vi "Main.vi"() -> ()   [LabVIEW 2014]
doc: "The myRIO Project template acquires acceleration data from the onboard accelerometer and displays the changes of acceleration values in a waveform chart."
uses:
  C:/Program Files (x86)/National Instruments/LabVIEW 2014/examples/robotics/Vision/Color Tracking/HueSlider.ctl
  <vilib>/myRIO/Instrument Drivers/Onboard IO/AI/typedefs/AI Reference.ctl
  <vilib>/myRIO/Common/Instrument Driver Framework/Utilities/typedefs/myRIO Generic Hardware Reference.ctl
  <vilib>/myRIO/Common/Instrument Driver Framework/Utilities/typedefs/Hardware Version Enum.ctl
  <vilib>/myRIO/Common/Instrument Driver Framework/Utilities/typedefs/myRIO v1.0 Reference.ctl
  <vilib>/myRIO/Common/Instrument Driver Framework/Utilities/typedefs/Generic FPGA Reference.ctl
  <vilib>/myRIO/Common/Instrument Driver Framework/myRIO v1.0/AI/typedefs/AI Channels List.ctl
  <vilib>/myRIO/Common/Instrument Driver Framework/myRIO v1.0/AI/typedefs/AI Channels Enum.ctl
  <vilib>/myRIO/Common/Instrument Driver Framework/Utilities/typedefs/Analog Scaling Constants List.ctl
  <vilib>/myRIO/Common/Instrument Driver Framework/Utilities/typedefs/Analog Scaling Constants.ctl
  <vilib>/userdefined/High Color/nirio_resource_hc.ctl
  <vilib>/myRIO/Instrument Drivers/Onboard IO/PWM/typedefs/PWM Reference.ctl
  <vilib>/myRIO/Common/Instrument Driver Framework/myRIO v1.0/PWM/typedefs/PWM Channels Enum.ctl
  <vilib>/myRIO/Instrument Drivers/Onboard IO/PWM/typedefs/PWM Configuration.ctl
  <vilib>/myRIO/Instrument Drivers/Onboard IO/DIO/typedefs/DIO Reference.ctl
  <vilib>/myRIO/Common/Instrument Driver Framework/myRIO v1.0/DIO/typedefs/DIO Channels List.ctl
  <vilib>/myRIO/Common/Instrument Driver Framework/myRIO v1.0/DIO/typedefs/DIO Channels Enum.ctl
  <vilib>/myRIO/Common/Instrument Driver Framework/myRIO v1.0/Encoder/typedefs/Encoder Signal Mode.ctl
  <vilib>/myRIO/Instrument Drivers/Onboard IO/Encoder/typedefs/Encoder Reference.ctl
  <vilib>/myRIO/Common/Instrument Driver Framework/myRIO v1.0/Encoder/typedefs/Encoder Channels Enum.ctl
  <vilib>/myRIO/Common/Instrument Driver Framework/myRIO v1.0/Encoder/typedefs/Encoder Configuration v1.0.ctl
  <vilib>/myRIO/Common/Instrument Driver Framework/Utilities/vis/Is FPGA Ref Available.vi
  <vilib>/myRIO/Common/Instrument Driver Framework/myRIO v1.0/AI/vis/myRIO v1.1 Open AI.vi
  <vilib>/myRIO/Instrument Drivers/Onboard IO/AI/vis/Read.vi
  <vilib>/myRIO/Common/Instrument Driver Framework/myRIO v1.0/PWM/vis/myRIO v1.1 Open PWM.vi
  <vilib>/myRIO/Instrument Drivers/Onboard IO/PWM/vis/Set Duty Cycle and Frequency.vi
  <vilib>/myRIO/Common/Instrument Driver Framework/myRIO v1.0/Encoder/vis/myRIO v1.1 Open Encoder.vi
  <vilib>/myRIO/Instrument Drivers/Onboard IO/Encoder/vis/Read.vi
  <vilib>/myRIO/Common/Instrument Driver Framework/myRIO v1.0/DIO/vis/myRIO v1.1 Open DIO.vi
  <vilib>/myRIO/Instrument Drivers/Onboard IO/DIO/vis/Write.vi
  <vilib>/myRIO/Common/Instrument Driver Framework/Utilities/vis/Validate Channels.vi
  <vilib>/myRIO/Common/Instrument Driver Framework/myRIO v1.0/AI/vis/myRIO v1.0 Reserve AI.vi
  <vilib>/myRIO/Common/Instrument Driver Framework/myRIO v1.0/PWM/vis/myRIO v1.0 Reserve PWM.vi
  <vilib>/myRIO/Common/Instrument Driver Framework/myRIO v1.0/Encoder/vis/myRIO v1.0 Reserve Encoder.vi
  <vilib>/myRIO/Common/Instrument Driver Framework/myRIO v1.0/DIO/vis/myRIO v1.0 Reserve DIO.vi
  <vilib>/myRIO/Common/Instrument Driver Framework/myRIO v1.0/UART/vis/myRIO v1.0 Close UART.vi
  <vilib>/myRIO/Common/Instrument Driver Framework/myRIO v1.0/AI/vis/myRIO v1.0 Build MUX Configuration AI.vi
  <vilib>/myRIO/Common/Instrument Driver Framework/myRIO v1.0/Resource Manager/vis/myRIO v1.0 Reserve Channel List.vi
  <vilib>/myRIO/Common/Instrument Driver Framework/myRIO v1.0/PWM/vis/myRIO v1.0 Build MUX Configuration PWM.vi
  <vilib>/myRIO/Common/Instrument Driver Framework/myRIO v1.0/Encoder/vis/myRIO v1.0 Build MUX Configuration Encoder.vi
  <vilib>/myRIO/Common/Instrument Driver Framework/myRIO v1.0/DIO/vis/myRIO v1.0 Build MUX Configuration DIO.vi
  <vilib>/myRIO/Common/Instrument Driver Framework/myRIO v1.0/Resource Manager/vis/myRIO v1.0 Reserve Channel.vi
  <vilib>/myRIO/Common/Instrument Driver Framework/myRIO v1.0/Resource Manager/vis/myRIO v1.0 Unreserve Channel.vi
  <vilib>/myRIO/Common/Instrument Driver Framework/myRIO v1.0/Resource Manager/vis/myRIO v1.0 Create Configuration List.vi
  <vilib>/myRIO/Common/Instrument Driver Framework/myRIO v1.0/Resource Manager/vis/myRIO v1.0 Build Mutex Name.vi
  <vilib>/Utility/VariantDataType/GetNumericInfo.vi
  <vilib>/Utility/error.llb/Error Cluster From Error Code.vi
  <vilib>/myRIO/Common/Instrument Driver Framework/myRIO v1.0/myRIO v1.1 Open.vi
  <vilib>/myRIO/Common/Instrument Driver Framework/myRIO v1.0/AI/vis/myRIO v1.0 Get Scaling Constants AI.vi
  <vilib>/myRIO/Common/Instrument Driver Framework/Utilities/vis/IO Manager.vi
  <vilib>/myRIO/Common/Instrument Driver Framework/Utilities/vis/Configuration Manager.vi
  <vilib>/myRIO/Common/Instrument Driver Framework/myRIO v1.0/myRIO v1.0 Close.vi
  <vilib>/myRIO/Common/Instrument Driver Framework/myRIO v1.0/AI/vis/myRIO v1.0 Read AI.vi
  <vilib>/myRIO/Common/Instrument Driver Framework/myRIO v1.0/Resource Manager/vis/myRIO v1.0 Configure IO.vi
  <vilib>/myRIO/Common/Instrument Driver Framework/myRIO v1.0/PWM/vis/myRIO v1.0 Write PWM.vi
  <vilib>/myRIO/Common/Instrument Driver Framework/myRIO v1.0/DIO/vis/myRIO v1.0 Write DIO.vi
  <vilib>/myRIO/Common/Instrument Driver Framework/myRIO v1.0/Encoder/vis/myRIO v1.0 Configure Encoder.vi
  <vilib>/myRIO/Common/Instrument Driver Framework/myRIO v1.0/Encoder/vis/myRIO v1.0 Read Encoder.vi
  <vilib>/myRIO/Common/Instrument Driver Framework/Utilities/vis/FPGA Ref Manager.vi
  <vilib>/myRIO/Common/Instrument Driver Framework/myRIO v1.0/myRIO v1.0 Reset FPGA.vi
  <vilib>/myRIO/Common/Instrument Driver Framework/myRIO v1.0/IRQ/vis/myRIO v1.0 IRQ Info FGV.vi
  <vilib>/myRIO/Common/Instrument Driver Framework/myRIO v1.0/IRQ/vis/myRIO v1.0 Timer IRQ Info FGV.vi
  <vilib>/myRIO/Common/Instrument Driver Framework/myRIO v1.0/IRQ/vis/myRIO v1.0 ISR Agent.vi
  <vilib>/myRIO/Express VI/Onboard IO/AI/AI Express VI.xnode
  <vilib>/myRIO/Instrument Drivers/Onboard IO/AI/vis/myRIO AI Open.xnode
  <vilib>/myRIO/Express VI/Onboard IO/PWM/PWM Express VI.xnode
  <vilib>/myRIO/Instrument Drivers/Onboard IO/PWM/vis/myRIO PWM Open.xnode
  <vilib>/myRIO/Express VI/Onboard IO/DO/DO Express VI.xnode
  <vilib>/myRIO/Instrument Drivers/Onboard IO/DIO/vis/myRIO DIO Open.xnode
  <vilib>/myRIO/Express VI/Onboard IO/Encoder/Encoder Express VI.xnode
  <vilib>/myRIO/Instrument Drivers/Onboard IO/Encoder/vis/myRIO Encoder Open.xnode
  <vilib>/myRIO/Instrument Drivers/Utilities/Utilities.lvlib
  <vilib>/myRIO/Instrument Drivers/Onboard IO/PWM/PWM.lvlib
  <vilib>/myRIO/Instrument Drivers/Onboard IO/DIO/DIO.lvlib
  <vilib>/myRIO/Instrument Drivers/Onboard IO/Encoder/Encoder.lvlib
  <vilib>/vision/driver/NI_Vision_Acquisition_Software.lvlib
  <vilib>/vision/NI_Vision_Development_Module.lvlib
  <vilib>/myRIO/Instrument Drivers/Onboard IO/AI/AI.lvlib
  <vilib>/Analysis/NI_AALPro.lvlib
  <vilib>/Analysis/NI_AALBase.lvlib
panel:
  out "LCD display":string
  in  "Samples":i32=128
  in  "Amplitude":dbl=5.0 format="%#.6g"
  in  "Width (samples)":i32=32
  in  "Delay (samples)":i32=64
  in  "Filter rank":i32(slide)=7 scale=0.0..30.0
  in  "Gaussian noise sigma":dbl(slide)=0.8 scale=0.0..2.0
  out "Waveform Graph":dbl[][](graph)
  out "Width (est)":dbl format="%#.2g"
  out "Delay (est)":dbl format="%#.2g"
  out "Amplitude (est)":dbl format="%#.2g"
  in  "seed":i32=-1
  out "Gauss 1 fit":cluster{"a":dbl, "m":dbl, "sigma":dbl}
  out "Gauss 2 fit":cluster{"a":dbl, "m":dbl, "sigma":dbl}
  out "Gauss 3 fit":cluster{"a":dbl, "m":dbl, "sigma":dbl}
  out "DC offset fit":dbl
  out "웨이브폼 차트":dbl(graph)
  out "C/AI0 (C/AI0 (AI0))":dbl
  out "Image 2":T1(plugin-control)
  in  "Speed\n(PWM Duty %) 2":dbl(slide)=1.0
  in  "Hue range":T2={"Min"=232, "Max"=21} scale=0.0..255.0
  in  "Stop 2":bool
  out "Image":T1(plugin-control)
  in  "Camera Name":refnum<k21>="cam3" caption="IMAQdx Session"
  in  "Reset Counter":bool
  out "Counter Value":i32
  out "Counter Direction":enum16{"Counting Up", "Counting Down"}(ring)
  in  "Direction":bool
  in  "Speed\n(PWM Duty %)":dbl(slide)=1.0
  out "error out":errorcluster
  in  "Stop":bool
  # "Control Motor"
  # "Read Encoder"
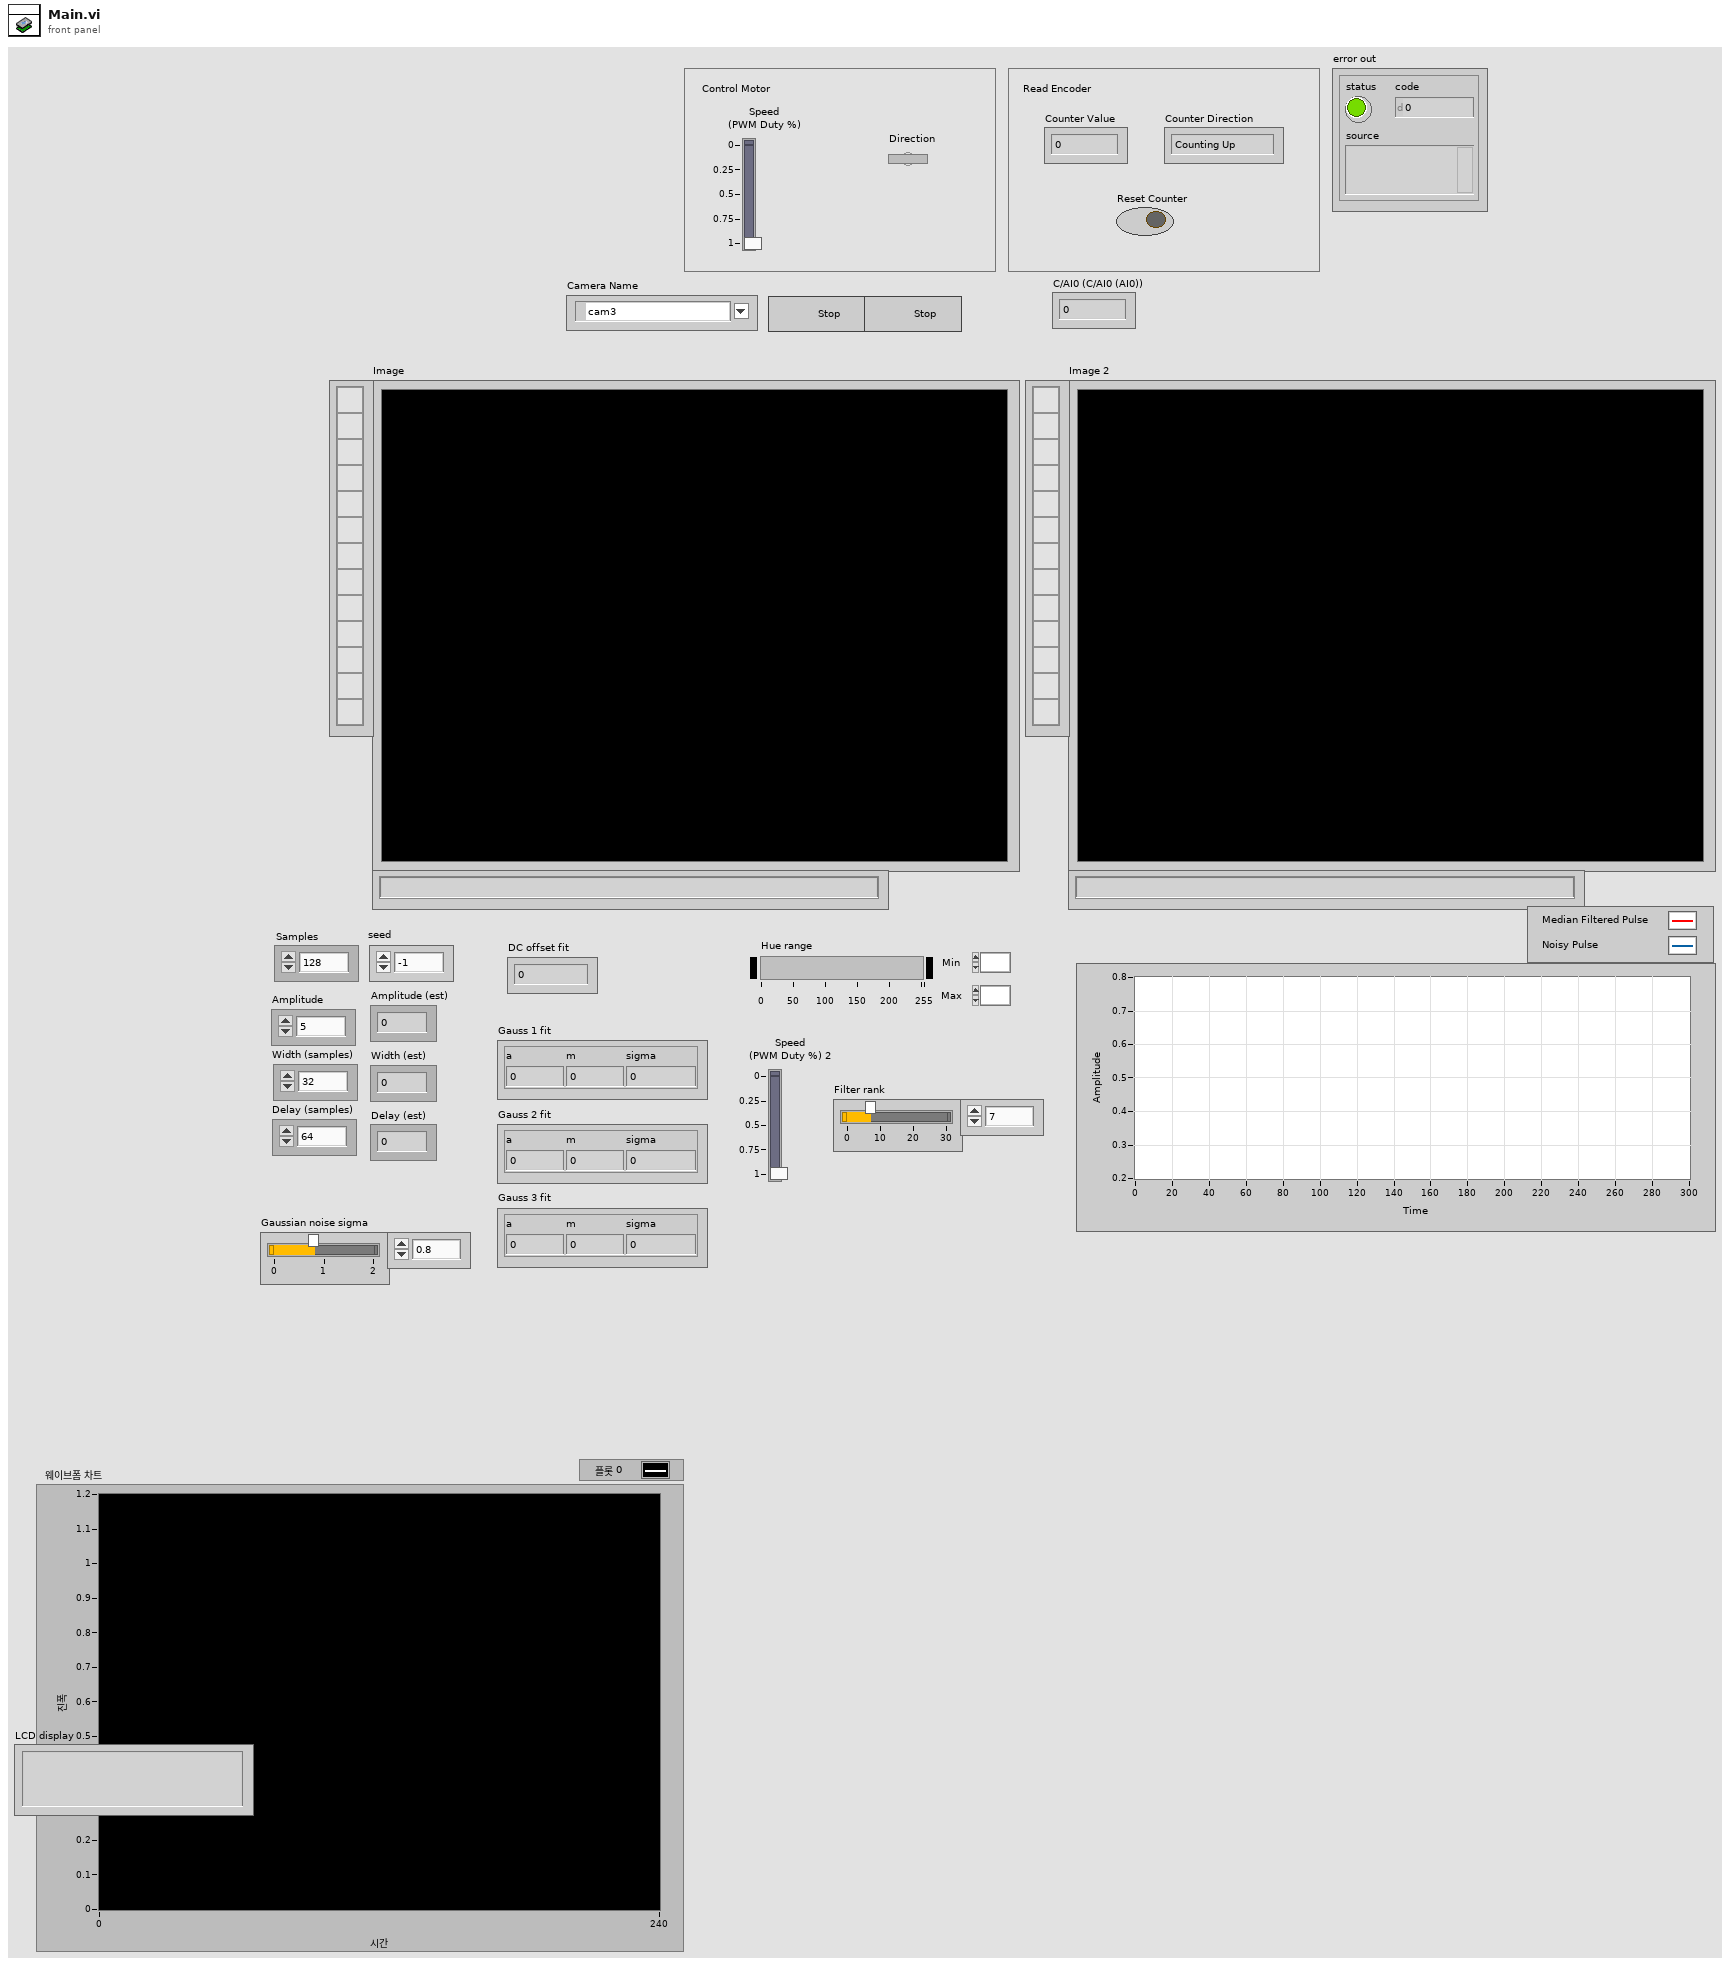
[diagram p1: front panel]
types:
  T1 = typedef "IMAQ Image.ctl" = refnum<image>
  T2 = typedef "HueSlider.ctl" = cluster{"Min":i32, "Max":i32}
  T3 = typedef "IMAQ Circle" = cluster{"Center X":i32, "Center Y":i32, "Inner Radius":i32, "Outer Radius":i32, "Start Angle":dbl, "End Angle":dbl}
  T4 = typedef "AI.lvlib/AI Reference.ctl" = cluster{"myRIO Reference":T5, "AI Channels List":T9, "AI Scaling Constants List":T11}
  T5 = typedef "myRIO Generic Hardware Reference.ctl" = cluster{"myRIO Model":T6, "myRIO Hardware Reference":T7}
  T6 = typedef "Hardware Version Enum.ctl" = enum16{"Unknown", "myRIO-1900", "myRIO-1950"}
  T7 = typedef "myRIO v1.0 Reference.ctl" = cluster{"Generic FPGA Reference":T8, "Allow multiple opens":bool}
  T8 = typedef "Generic FPGA Reference.ctl" = refnum<k20>
  T9 = typedef "AI Channels List.ctl" = T10[]
  T10 = typedef "AI Channels Enum.ctl" = enum16{"Not Connected", "AudioIn/Left", "AudioIn/Right", "C/AI0", "C/AI1", "A/AI0", "A/AI1", "A/AI2", "A/AI3", "B/AI0", "B/AI1", "B/AI2", "B/AI3"}
  T11 = typedef "Analog Scaling Constants List.ctl" = T12[]
  T12 = typedef "Analog Scaling Constants.ctl" = cluster{"LSB Weight (Volts)":dbl, "Offset (Volts)":dbl, "Signed?":bool}
  T13 = typedef "nirio_resource_hc.ctl" = tag
  T14 = typedef "IMAQ Rectangle" = cluster{"Left":i32, "Top":i32, "Right":i32, "Bottom":i32, "Rotation":dbl}
  T15 = typedef "PWM.lvlib/PWM Reference.ctl" = cluster{"myRIO Reference":T5, "PWM Channels Enum":T16, "PWM Configuration":T17}
  T16 = typedef "PWM Channels Enum.ctl" = enum16{"Not Connected", "C/PWM0", "C/PWM1", "A/PWM0", "A/PWM1", "A/PWM2", "B/PWM0", "B/PWM1", "B/PWM2"}
  T17 = typedef "PWM.lvlib/PWM Configuration.ctl" = cluster{"Frequency":dbl, "Duty Cycle":dbl}
  T18 = typedef "Encoder.lvlib/Encoder Reference.ctl" = cluster{"myRIO Reference":T5, "Encoder Channels Enum":T19}
  T19 = typedef "Encoder Channels Enum.ctl" = enum16{"Not Connected", "C/ENC0", "C/ENC1", "A/ENC", "B/ENC"}
  T20 = typedef "Encoder Signal Mode.ctl" = enum16{"Quadrature phase signal", "Step and direction signal"}
  T21 = typedef "DIO.lvlib/DIO Reference.ctl" = cluster{"myRIO Reference":T5, "DIO Channels List":T22}
  T22 = typedef "DIO Channels List.ctl" = T23[]
  T23 = typedef "DIO Channels Enum.ctl" = enum16{"Not Connected", "C/DIO0", "C/DIO1", "C/DIO2", "C/DIO3", "C/DIO4", "C/DIO5", "C/DIO6", "C/DIO7", "A/DIO0", "A/DIO1", "A/DIO2", "A/DIO3", "A/DIO4", "A/DIO5", "A/DIO6", "A/DIO7", "A/DIO8", "A/DIO9", "A/DIO10", "A/DIO11", "A/DIO12", "A/DIO13", "A/DIO14", "A/DIO15", "B/DIO0", "B/DIO1", "B/DIO2", "B/DIO3", "B/DIO4", "B/DIO5", "B/DIO6", "B/DIO7", "B/DIO8", "B/DIO9", "B/DIO10", "B/DIO11", "B/DIO12", "B/DIO13", "B/DIO14", "B/DIO15", "LED0", "LED1", "LED2", "LED3", "Button0"}
  T24 = typedef "IMAQdx.ctl" = refnum<k21>
  T25 = cluster{"Global Rectangle":i32[], "Contours":cluster{"Contour Type":u32, "ROI Type":u32, "Points":i32[]}[]}
  T26 = cluster{"Center":cluster{"X":sgl, "Y":sgl}, "Radius":dbl}
  T27 = typedef "ROI Descriptor" = cluster{"Global Rectangle":i32[], "Contours":cluster{"ID":enum32{"External", "Internal"}, "Type":u32, "Coordinates":i32[]}[]}
  T28 = cluster{"Area":dbl, "Number of Holes":dbl, "Bounding Rect":cluster{"Left":dbl, "Top":dbl, "Right":dbl, "Bottom":dbl}, "Center of Mass":cluster{"X":dbl, "Y":dbl}, "Orientation":dbl, "Dimensions":cluster{"Width":dbl, "Height":dbl}}[]
  T29 = cluster{"Left":dbl, "Top":dbl, "Right":dbl, "Bottom":dbl}
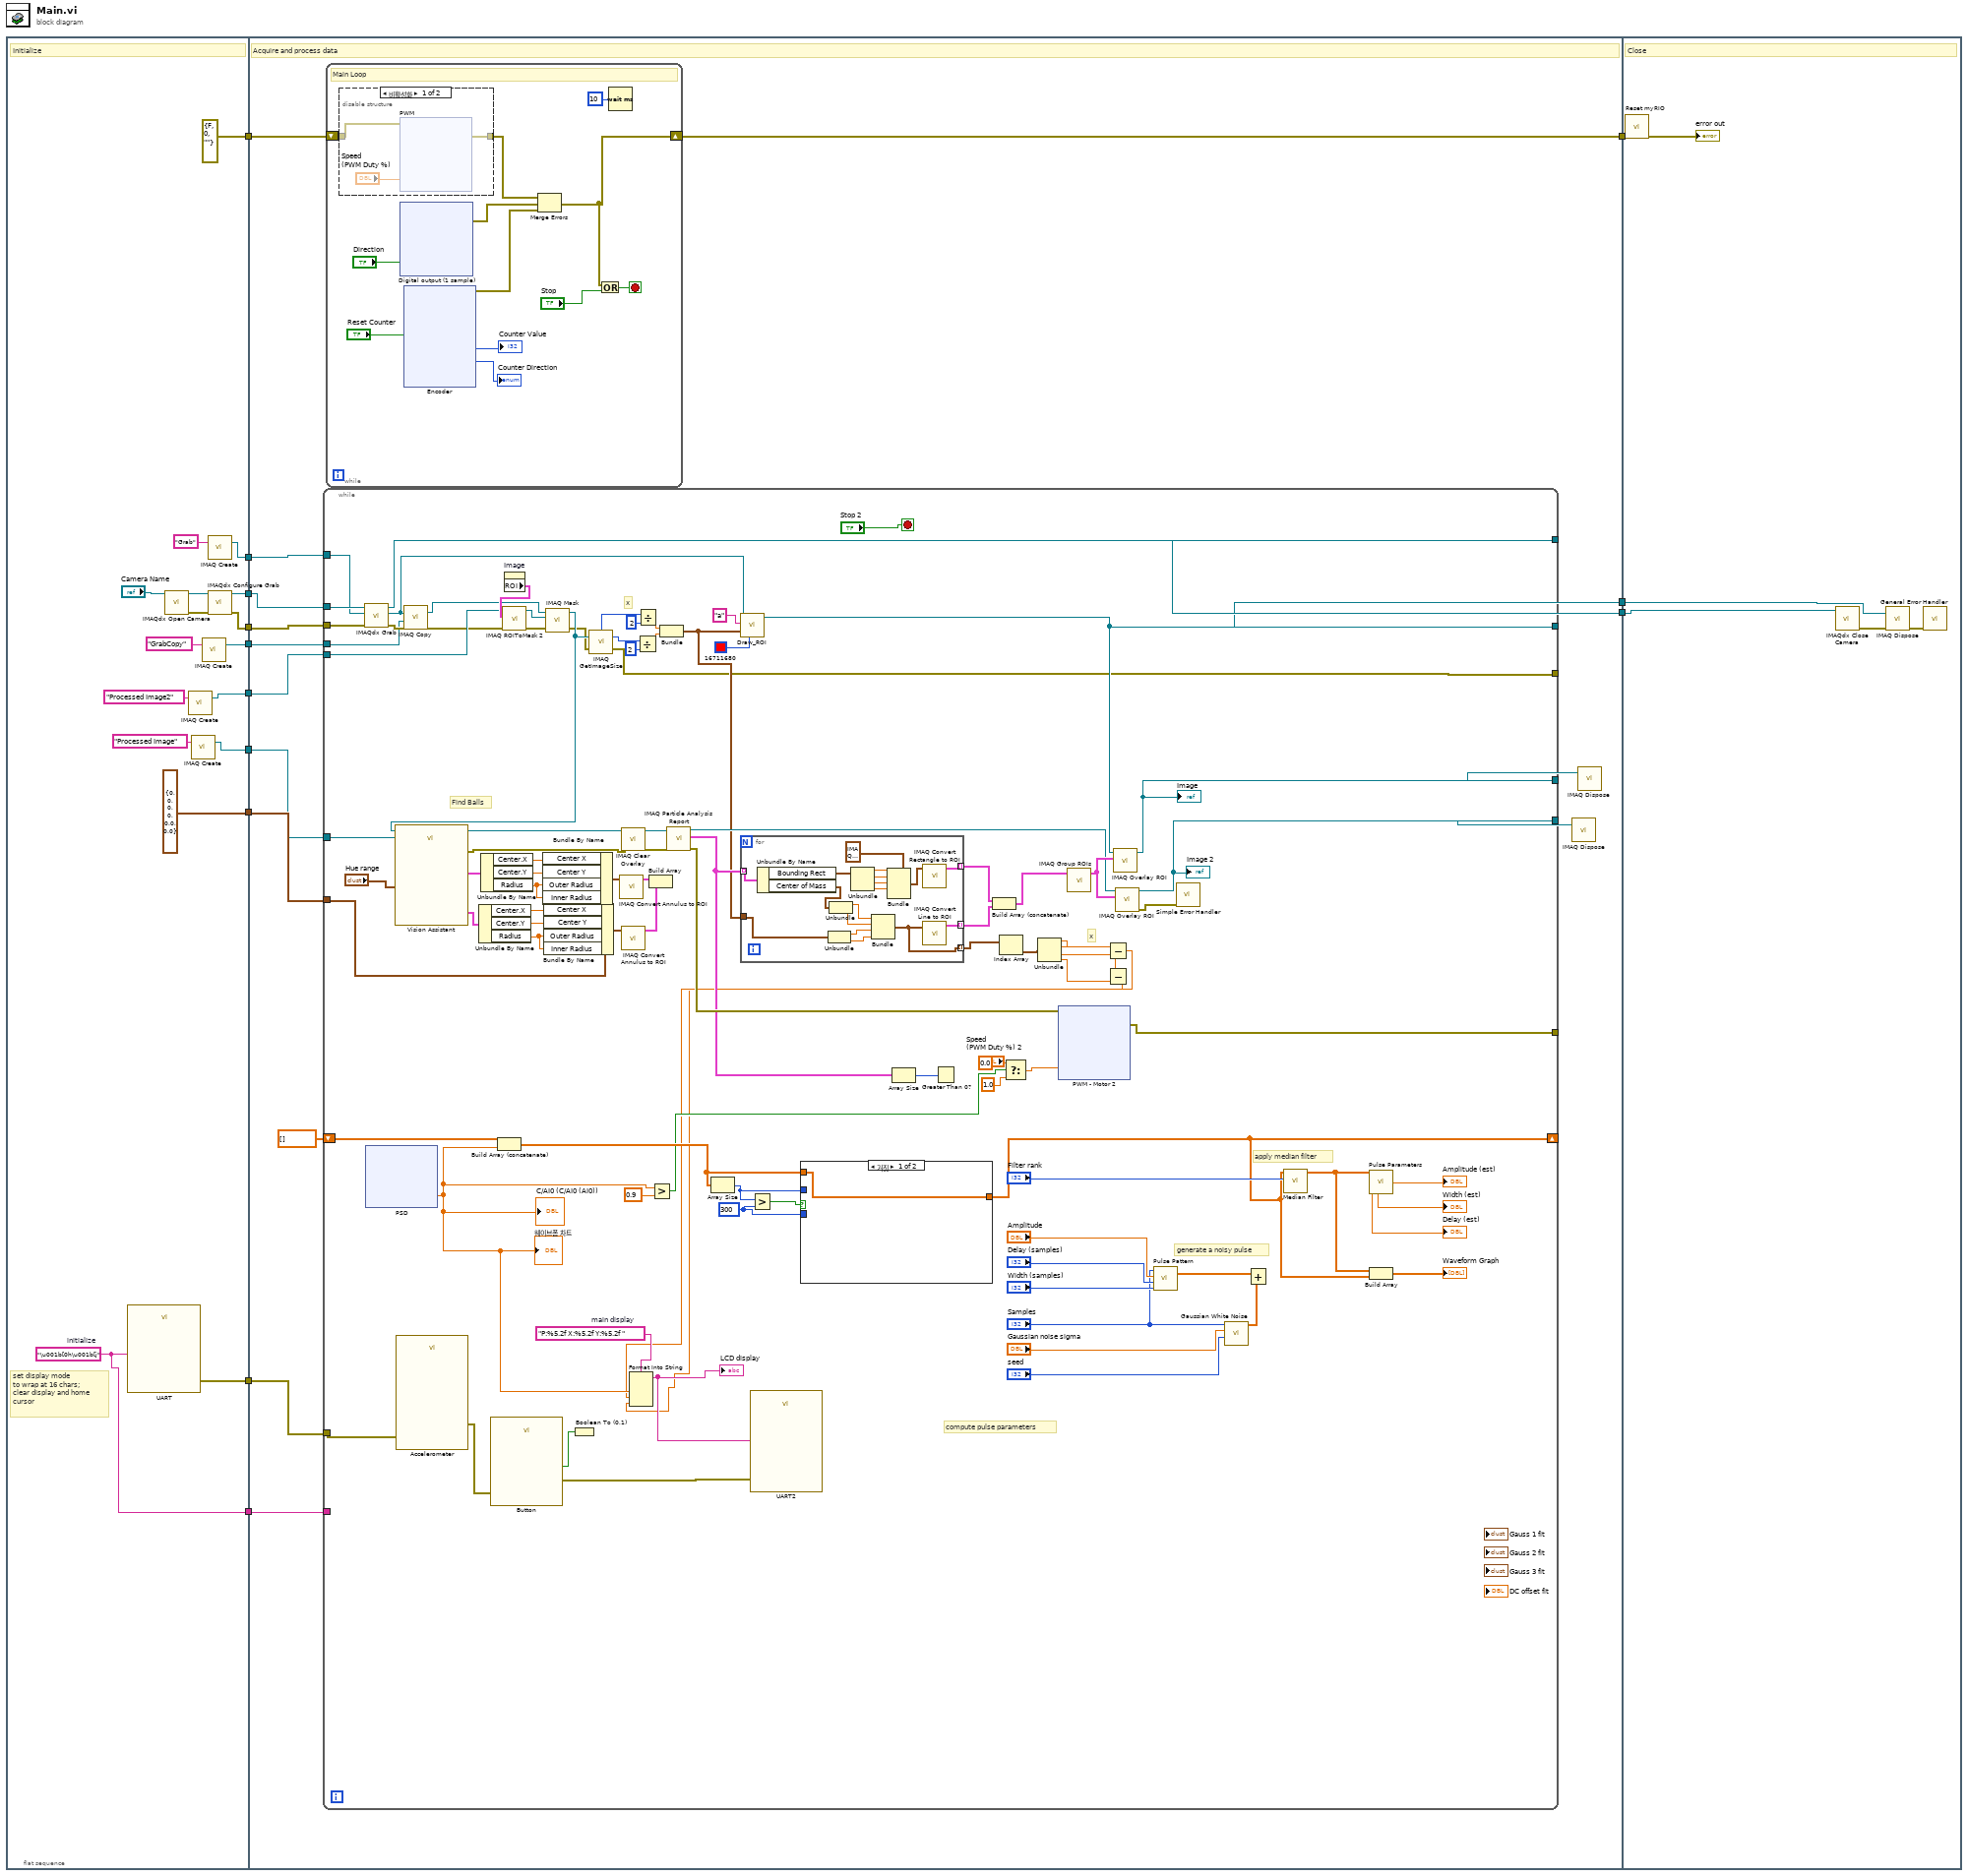
[diagram p0: block diagram]
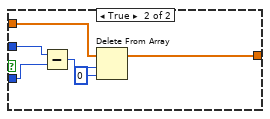
[diagram p2: hidden frame]
diagram:
  n1 = flat-sequence {
    tunnel: [errorcluster {"status"=FALSE, "code"=0, "source"=""} ("error in (no error)")] -> w13
    tunnel: [w25] -> w11
    tunnel: [w24] -> w10
    tunnel: [w23] -> w9
    tunnel: [T3 {"Center X"=0, "Center Y"=0, "Inner Radius"=0, "Outer Radius"=0, "Start Angle"=0.0, "End Angle"=0.0} ("Annulus")] -> w6
    tunnel: [w20] -> w5
    tunnel: [w18] -> w4
    tunnel: [w16] -> w3
    tunnel: [w15] -> w2
    tunnel: [w14] -> w1
    tunnel: w13 -> [w46]
    tunnel: [w45] -> w12
    tunnel: w11 -> [w44]
    tunnel: w10 -> [w43]
    tunnel: w9 -> [w42]
    tunnel: [w34] -> w8
    tunnel: [w41] -> w7
    tunnel: w6 -> [w40]
    tunnel: w5 -> [w39]
    tunnel: w4 -> [w36]
    tunnel: w3 -> [w35]
    tunnel: w2 -> [w32]
    tunnel: w1 -> [w31]
    tunnel: w12 -> [w377]
    tunnel: w8 -> [w373]
    tunnel: w7 -> [w372]
    frame #0 {
      w14 = "\u001b[0h\u001b[j"  # initialize
      # "set display mode\nto wrap at 16 chars;\nclear display and home\ncursor"
      # "Initialize"
      n2 = call "UART"("Characters to Write"=w14) -> ("error out"=w15:errorcluster)  [unwired: 25 in, 1 out]
      n3 = call <vilib>:"IMAQdx Open Camera.vi"("Session In"="Camera Name") -> ("error out"=w29:errorcluster, "Session Out"=w28:T24)  [unwired: 2 in, 7 out]
      n4 = call "IMAQ Create"("Image Name"="Processed Image2") -> ("New Image"=w18:T1)  [unwired: 3 in, 2 out]
      n5 = call "IMAQ Create"("Image Name"="Processed Image") -> ("New Image"=w20:T1)  [unwired: 3 in, 2 out]
      n6 = call "IMAQ Create"("Image Name"="GrabCopy") -> ("New Image"=w16:T1)  [unwired: 3 in, 2 out]
      n7 = call "IMAQ Create"("Image Name"="Grab") -> ("New Image"=w25:T1)  [unwired: 3 in, 2 out]
      n8 = call <vilib>:"IMAQdx Configure Grab.vi"("error in"=w29, "Session In"=w28) -> ("error out"=w23:errorcluster, "Session Out"=w24:T24)  [unwired: 8 out]
    }
    frame #1 {
      # "Acquire and process data"
      n9 = while {
        tunnel: [w141] -> w41
        tunnel: w42 -> [w143]
        tunnel: w43 -> [w144]
        tunnel: w44 -> [w142]
        tunnel: w40 -> [w123]
        tunnel: w39 -> [w122]
        tunnel: [w121] -> _
        tunnel: [w88] -> w38
        tunnel: [w87] -> w37
        tunnel: w36 -> [w111]
        tunnel: w35 -> [w96]
        tunnel: [w89] -> w34
        shift-right: [w66] -> _
        shift-left: dbl[] [] -> [w85]
        tunnel: [w63] -> _
        tunnel: w32 -> [w59]
        tunnel: w31 -> [_]
        stop <- "Stop 2" stop-if-true
        w51 = "P:%5.2f X:%5.2f Y:%5.2f "  # main display
        w82 = 300 ("y")
        # "x"
        # "generate a noisy pulse"
        # "apply median filter"
        # "compute pulse parameters"
        # "x"
        # "Find Balls"
        n10 = call <vilib>:"IMAQdx Grab.vi"("error in"=w143, "Image In"=w142, "Session In"=w144) -> ("error out"=w98:errorcluster, "Image Out"=w94:T1, "Session Out"=w141:T24)  [unwired: 1 in, 5 out]
        n11 = xnode "PSD"() -> ("C/AI0 (C/AI0 (AI0))"=w50:dbl)  [unwired: 1 in, 1 out]
        "C/AI0 (C/AI0 (AI0))" <- w50
        "웨이브폼 차트" <- w50
        n12 = call "Accelerometer"("error in (no error)"=w59) -> ("error out"=w60:errorcluster)  [unwired: 23 in, 3 out]
        n13 = call "IMAQ Copy"("error in (no error)"=w98, "Image Dst"=w96, "Image Src"=w94) -> ("error out"=w97:errorcluster, "Image Dst Out"=w95:T1)  [unwired: 3 in]
        n14 = call "Button"("error in (no error)"=w60) -> ("Value"=w61:bool, "error out"=w47:errorcluster)  [unwired: 25 in]
        n15 = Build Array (concatenate)(w85, w50) -> (w81:dbl[])
        n16 = property on="Image" class="ImageControl"() -> ("ROI"=w113:T25)  [unwired: 2 in, 2 out]
        n17 = call "IMAQ ROIToMask 2"("error in (no error)"=w97, "ROI Descriptor"=w113, "Image"=w111) -> ("error out"=w109:errorcluster, "Image Out"=w110:T1)  [unwired: 6 in, 1 out]
        n18 = call "IMAQ Mask"("error in (no error)"=w109, "Image Mask"=w110, "Image Src"=w95) -> ("error out"=w64:errorcluster, "Image Dst Out"=w93:T1)  [unwired: 2 in]
        n19 = call "Vision Assistant"("Image In"=w93, "Image Dst"=w122, "Red or Hue Range (Color Threshold)"="Hue range") -> ("Image Out"=w136:T1, "Best Circle (Fit Circle Ball 1)"=w124:T26, "Best Circle (Fit Circle Ball 2)"=w133:T26, "error out"=w138:errorcluster)  [unwired: 1 in, 20 out]
        n20 = Unbundle By Name(w133) -> ("Center.X"=w127:sgl, "Center.Y"=w128:sgl, "Radius"=w134:dbl)
        n21 = Unbundle By Name(w124) -> ("Center.X"=w125:sgl, "Center.Y"=w126:sgl, "Radius"=w135:dbl)
        n22 = Bundle By Name(cluster=w123, "Center X"=w125, "Center Y"=w126, "Outer Radius"=w135, "Inner Radius"=w135) -> (w129:T3)
        n23 = Bundle By Name(cluster=w123, "Center X"=w127, "Center Y"=w128, "Outer Radius"=w134, "Inner Radius"=w134) -> (w130:T3)
        n24 = Boolean To (0,1)(Boolean=w61) -> ()  [unwired: 1 out]
        n25 = call "IMAQ GetImageSize"("Image"=w93, "error in (no error)"=w64) -> ("Y Resolution"=w103:i32, "X Resolution"=w106:i32, "error out"=w63:errorcluster)  [unwired: 2 in]
        n26 = call "IMAQ Convert Annulus to ROI"("Annulus"=w129) -> ("ROI Descriptor"=w131:T27)  [unwired: 1 in, 8 out]
        n27 = call "IMAQ Clear Overlay"("error in (no error)"=w138, "Image"=w136) -> ("error out"=w107:errorcluster, "Image Out"=w116:T1)  [unwired: 1 in, 7 out]
        n28 = call "IMAQ Convert Annulus to ROI"("Annulus"=w130) -> ("ROI Descriptor"=w132:T27)  [unwired: 1 in, 8 out]
        n29 = Divide(x=w103, y=2) -> (x/y=w101:dbl)
        n30 = Divide(x=w106, y=2) -> (x/y=w102:dbl)
        n31 = Build Array(w131, w132) -> ()  [unwired: 1 out]
        n32 = Greater?(x=w50, y=0.9) -> (0:w65:bool)
        n33 = Bundle(w102, w101) -> (w92:cluster{dbl, dbl})  [unwired: 1 in]
        n34 = call "IMAQ Particle Analysis Report"("error in (no error)"=w107, "Image"=w116) -> ("error out"=w114:errorcluster, "Particle Reports (Pixels)"=w108:T28, "Image Out (duplicate)"=w115:T1)  [unwired: 4 in, 3 out]
        n35 = Array Size(array=w81) -> (size(s)=w83:i32)
        n36 = call "Draw_ROI.vi"("Color"=u32 16711680, "클러스터"=w92, "Group"="a", "참조 번호 입력"=w94) -> ("참조 번호 출력"=w89:T1)  [unwired: 7 in]
        n37 = for {
          tunnel: w108 -> [w205] mode=indexing
          tunnel: [w197] -> w91 mode=indexing
          tunnel: w92 -> [w193]
          tunnel: [w190] -> w58 mode=indexing
          tunnel: [w189] -> w57 mode=indexing
          n38 = Unbundle By Name(w205) -> ("Bounding Rect"=w203:T29, "Center of Mass"=w196:cluster{"X":dbl, "Y":dbl})
          n39 = Unbundle(w193) -> (w192:dbl, w191:dbl)
          n40 = Unbundle(w196) -> ("X"=w195:dbl, "Y"=w194:dbl)
          n41 = Unbundle(w203) -> ("Left"=w202:dbl, "Top"=w201:dbl, "Right"=w200:dbl, "Bottom"=w199:dbl)
          n42 = Bundle("X"=w195, "Y"=w194, w192, w191) -> (w189:cluster{"X":dbl, "Y":dbl, dbl, dbl})  [unwired: 1 in]
          n43 = Bundle(cluster=T14 {"Left"=0, "Top"=0, "Right"=0, "Bottom"=0, "Rotation"=0.0} ("Rectangle"), "Left"=w202, "Top"=w201, "Right"=w200, "Bottom"=w199) -> (w198:T14)  [unwired: 1 in]
          n44 = call "IMAQ Convert Rectangle to ROI"("Rectangle"=w198) -> ("ROI Descriptor"=w197:T27)  [unwired: 8 in, 1 out]
          n45 = call "IMAQ Convert Line to ROI"("Line"=w189) -> ("ROI Descriptor"=w190:T27)  [unwired: 8 in, 1 out]
        }
        n46 = Greater?(x=w83, y=w82) -> (0:w84:bool)
        n47 = case shown="거짓" w84 {
          tunnel: w81 -> [w145 w151]
          tunnel: w83 -> [_ w150]
          tunnel: w82 -> [_ w149]
          tunnel: [w145 w146] -> w66
          frame False {
          }
          frame True {
            n48 = Subtract(x=w150, y=w149) -> (x-y=w148:i32)
            n49 = Delete From Array(array=w151, length=w148, index=0 ("인덱스")) -> (array with subset deleted=w146:dbl[])  [unwired: 1 out]
          }
        }
        n50 = Array Size(array=w108) -> (size(s)=w120:i32)
        n51 = Greater Than 0?(x=w120) -> ()  [unwired: 1 out]
        n52 = Build Array (concatenate)(w91, w58) -> (w90:T27[])
        n53 = Index Array(array=w57) -> (element=w56:cluster{"X":dbl, "Y":dbl, dbl, dbl})  [unwired: 1 in]
        n54 = Select(t=0.0, s=w65, f=1.0) -> (s? t:f=w117:dbl)
        n55 = Unbundle(w56) -> ("X"=w55:dbl, "Y"=w53:dbl, w54:dbl, w52:dbl)
        n56 = xnode "PWM - Motor 2"("Duty Cycle"=w117, "error in (no error)"=w114) -> ("error out"=w121:errorcluster)
        n57 = call "IMAQ Group ROIs"("ROI Descriptors"=w90) -> ("ROI Descriptor out"=w137:T27)  [unwired: 1 in, 3 out]
        n58 = Subtract(x=w55, y=w54) -> (x-y=w49:dbl)
        n59 = Subtract(x=w53, y=w52) -> (x-y=w48:dbl)
        n60 = Format Into String "Format Into String"(format string=w51, w50, w49, w48) -> (resulting string=w62:string)  [unwired: 2 in, 1 out]
        "LCD display" <- w62
        n61 = call "UART2"("Characters to Write"=w62, "error in (no error)"=w47) -> ()  [unwired: 24 in, 2 out]
        n62 = call "IMAQ Overlay ROI"("ROI Descriptor"=w137, "Image"=w89) -> ("Image Out"=w88:T1)  [unwired: 4 in, 5 out]
        "Image" <- w88
        n63 = call "IMAQ Overlay ROI"("ROI Descriptor"=w137, "Image"=w115) -> ("error out"=w139:errorcluster, "Image Out"=w87:T1)  [unwired: 4 in, 4 out]
        "Image 2" <- w87
        n64 = call <vilib>:"Pulse Pattern.vi"("width"="Width (samples)", "delay"="Delay (samples)", "amplitude"="Amplitude", "samples"="Samples") -> ("Pulse Pattern"=w75:dbl[])  [unwired: 1 out]
        n65 = call <vilib>:"Simple Error Handler.vi"("error in (no error)"=w139) -> ()  [unwired: 1 in, 8 out]
        n66 = call <vilib>:"Gaussian White Noise.vi"("seed"="seed", "standard deviation"="Gaussian noise sigma", "samples"="Samples") -> ("Gaussian noise pattern"=w68:dbl[])  [unwired: 7 in, 1 out]
        n67 = Add(x=w75, y=w68) -> ()  [unwired: 1 out]
        n68 = call <vilib>:"Median Filter.vi"("left rank"="Filter rank", "X"=w66) -> ("Filtered X"=w80:dbl[])  [unwired: 8 in, 1 out]
        n69 = call <vilib>:"Pulse Parameters.vi"("X"=w80) -> ("amplitude"=→"Amplitude (est)":dbl, "delay"=→"Delay (est)":dbl, "duration"=→"Width (est)":dbl)  [unwired: 4 in, 8 out]
        n70 = Build Array(w80, w66) -> (→"Waveform Graph":dbl[][])
      }
      n71 = while {
        shift-right: [w246] -> w45
        shift-left: w46 -> [w249]
        stop <- w251 stop-if-true
        # "Main Loop"
        n72 = disable-structure shown="비활성화" {
          disable-tunnel: w249 -> [w254 _]
          disable-tunnel: [w253 _] -> w248
          frame Disabled {
            n73 = xnode "PWM"("Duty Cycle"="Speed\n(PWM Duty %)", "error in (no error)"=w254) -> ("error out"=w253:errorcluster)
          }
          frame Enabled {
          }
        }
        n74 = xnode "Digital output (1 sample)"("DIR0 (A/DIO6 (Pin 23))"="Direction") -> ("error out"=w247:errorcluster)  [unwired: 1 in]
        n75 = xnode "Encoder"("Reset Counter"="Reset Counter") -> ("Counter Value"=→"Counter Value":i32, "Counter Direction"=→"Counter Direction":enum16{"Counting Up", "Counting Down"}, "error out"=w242:errorcluster)  [unwired: 1 in, 1 out]
        n76 = Merge Errors(w248, w247, w242) -> (w246:errorcluster)
        n77 = Or(x=w246, y="Stop") -> (x .or. y?=w251:bool)
        n78 = Wait (ms)(milliseconds to wait=u32 10) -> ()  [unwired: 1 out]
      }
      n79 = call "IMAQ Dispose"("Image"=w37) -> ()  [unwired: 5 in, 1 out]
      n80 = call "IMAQ Dispose"("Image"=w38) -> ()  [unwired: 5 in, 1 out]
    }
    frame #2 {
      # "Close"
      n81 = call <vilib>:"Reset myRIO.vi"("error in (no error)"=w377) -> ("error out"=→"error out":errorcluster)  [unwired: 10 in]
      n82 = call <vilib>:"IMAQdx Close Camera.vi"("Session In"=w372) -> ("error out"=w375:errorcluster)  [unwired: 1 in, 9 out]
      n83 = call "IMAQ Dispose"("Image"=w373, "error in (no error)"=w375) -> ("error out"=w374:errorcluster)  [unwired: 4 in]
      n84 = call <vilib>:"General Error Handler.vi"("error in (no error)"=w374) -> ()  [unwired: 2 in, 13 out]
    }
  }
